vi "Drive for Distance.vi"(3 "Timeout (s)":dbl, 4 "Distance (m)":dbl, 5 "RobotDriveDevRef":T1={"DevStatus"={"status"=FALSE, "code"=0, "source"=""}, "Motors[]"=[], "Square Inputs"=FALSE, "Max Output"=1.0}) -> (2 "RobotDriveDevRef Out":T1={"DevStatus"={"status"=FALSE, "code"=0, "source"=""}, "Motors[]"=[], "Square Inputs"=FALSE, "Max Output"=1.0})   [LabVIEW 2016]
uses:
  <vilib>/Rock Robotics/WPI/RobotDrive/WPI_RobotDriveDevRef.ctl
  <vilib>/Rock Robotics/WPI/MotorControl/WPI_MotorControlDeviceRef.ctl
  <vilib>/Rock Robotics/WPI/MotorControl/WPI_MotorControlType.ctl
  <vilib>/Rock Robotics/SystemInterfaces/DIO/FPGA_DIOPWMChannel.ctl
  <vilib>/Rock Robotics/WPI/PWM/WPI_PWMDeadband.ctl
  <vilib>/Rock Robotics/Network Tables/NT Read Number.vi
  Robot Global Data.vi
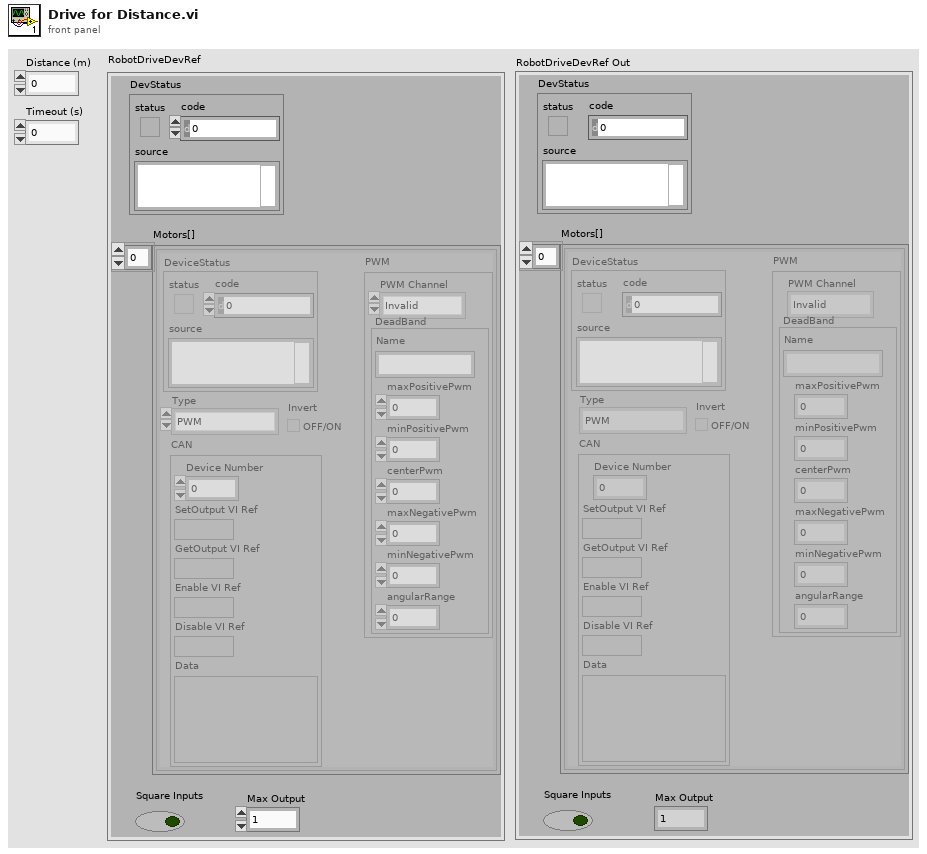
[diagram p1: front panel]
types:
  T1 = typedef "WPI_RobotDriveDevRef.ctl" = cluster{"DevStatus":errorcluster, "Motors[]":T2[], "Square Inputs":bool, "Max Output":dbl}
  T2 = typedef "WPI_MotorControlDeviceRef.ctl" = cluster{"DeviceStatus":errorcluster, "Type":T3, "PWM":cluster{"PWM Channel":T4, "DeadBand":T5}, "CAN":cluster{"Device Number":u8, "SetOutput VI Ref":variant, "GetOutput VI Ref":variant, "Enable VI Ref":variant, "Disable VI Ref":variant, "Data":variant}, "Invert":bool}
  T3 = typedef "WPI_MotorControlType.ctl" = enum16{"PWM", "CAN"}
  T4 = typedef "FPGA_DIOPWMChannel.ctl" = enum8{"PWM 0", "PWM 1", "PWM 2", "PWM 3", "PWM 4", "PWM 5", "PWM 6", "PWM 7", "PWM 8", "PWM 9", "PWM MXP 0", "PWM MXP 1", "PWM MXP 2", "PWM MXP 3", "PWM MXP 4", "PWM MXP 5", "PWM MXP 6", "PWM MXP 7", "PWM MXP 8", "PWM MXP 9", "Invalid"}
  T5 = typedef "WPI_PWMDeadband.ctl" = cluster{"Name":string, "maxPositivePwm":i32, "minPositivePwm":i32, "centerPwm":i32, "maxNegativePwm":i32, "minNegativePwm":i32, "angularRange":u16}
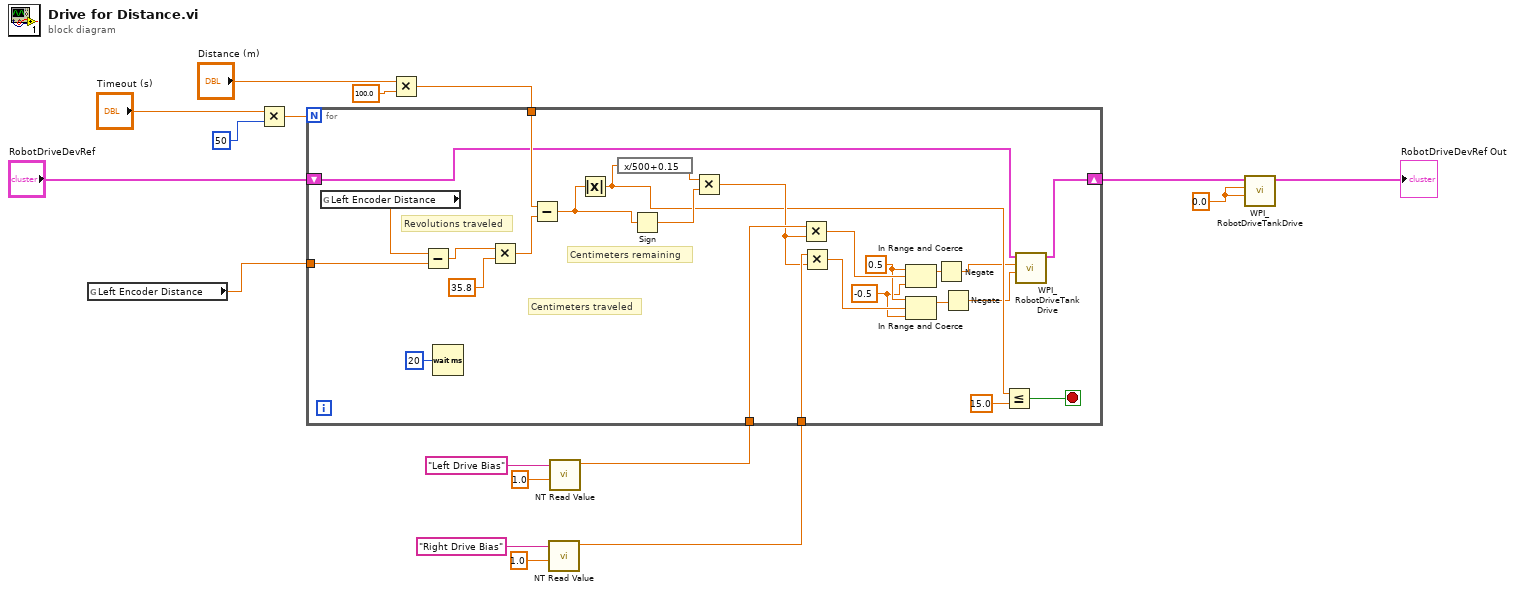
[diagram p0: block diagram]
diagram:
  w1 = 0.0 ("Left axis value")
  n1 = global read "Robot Global Data.vi" "Left Encoder Distance"() -> (w13:dbl)
  n2 = Multiply(x="Timeout (s)", y=50) -> (x*y=w5:dbl)
  n3 = Multiply(x="Distance (m)", y=100.0) -> (x*y=w10:dbl)
  n4 = call-poly <vilib>:"NT Read Value.vi"("Default Value"=1.0, "Name"="Right Drive Bias") -> ("Numeric"=w8:dbl)  [unwired: 8 in, 1 out]
  n5 = call-poly <vilib>:"NT Read Value.vi"("Default Value"=1.0, "Name"="Left Drive Bias") -> ("Numeric"=w9:dbl)  [unwired: 8 in, 1 out]
  n6 = for {
    N: w5 -> [_]
    tunnel: w13 -> [w42]
    tunnel: w10 -> [w41]
    tunnel: w9 -> [w34]
    tunnel: w8 -> [w33]
    shift-right: [w26] -> w3
    shift-left: "RobotDriveDevRef" -> [w27]
    stop <- w29 stop-if-true
    w22 = -0.5
    w23 = 0.5
    # "Centimeters remaining"
    # "Centimeters traveled"
    # "Revolutions traveled"
    n7 = global read "Robot Global Data.vi" "Left Encoder Distance"() -> (w43:dbl)
    n8 = Subtract(x=w43, y=w42) -> (x-y=w39:dbl)
    n9 = Wait (ms)(milliseconds to wait=u32 20) -> ()  [unwired: 1 out]
    n10 = Multiply(x=w39, y=35.8) -> (x*y=w38:dbl)
    n11 = Subtract(x=w41, y=w38) -> (x-y=w36:dbl)
    n12 = Absolute Value(x=w36) -> (abs(x)=w31:dbl)
    n13 = expression code="x/500+0.15"(w31) -> (w37:dbl)
    n14 = Sign(1:w36) -> (0:w35:dbl)
    n15 = Multiply(x=w37, y=w35) -> (x*y=w32:dbl)
    n16 = Multiply(x=w34, y=w32) -> (x*y=w25:dbl)
    n17 = Multiply(x=w33, y=w32) -> (x*y=w24:dbl)
    n18 = In Range and Coerce(upper limit=w23, x=w25, lower limit=w22) -> (coerced(x)=w21:dbl)  [unwired: 1 out]
    n19 = In Range and Coerce(upper limit=w23, x=w24, lower limit=w22) -> (coerced(x)=w19:dbl)  [unwired: 1 out]
    n20 = Negate(x=w21) -> (-x=w20:dbl)
    n21 = Negate(x=w19) -> (-x=w18:dbl)
    n22 = Less Or Equal?(x=w31, y=15.0) -> (x <= y?=w29:bool)
    n23 = call <vilib>:"WPI_RobotDriveTankDrive.vi"("Right axis value"=w18, "Left axis value"=w20, "RobotDriveDevRef"=w27) -> ("RobotDriveDevRef"=w26:T1)  [unwired: 6 in, 2 out]
  }
  n24 = call <vilib>:"WPI_RobotDriveTankDrive.vi"("Right axis value"=w1, "Left axis value"=w1, "RobotDriveDevRef"=w3) -> ("RobotDriveDevRef"=→"RobotDriveDevRef Out":T1)  [unwired: 6 in, 2 out]
